vi "FPGA Toggle FPGA LED.vi"() -> ()   [LabVIEW 2011]
uses:
  <vilib>/rvi/eio/common/nirviEmuTemplateMethod_errors.vi
  <vilib>/eio/EIONode/EIONode.xnode
panel:
  in  "FPGA LED period (ms)":u32=500
  out "FPGA LED":bool
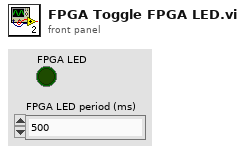
[diagram p1: front panel]
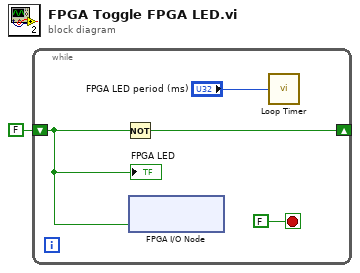
[diagram p0: block diagram]
diagram:
  n1 = while {
    shift-right: [w2] -> _
    shift-left: FALSE -> [w5]
    stop <- FALSE stop-if-true
    n2 = Not(x=w5) -> (.not. x?=w2:bool)
    n3 = xnode "FPGA I/O Node"("FPGA LED"=w5) -> ()  [unwired: 1 in, 1 out]
    n4 = call "Loop Timer"("Count(mSec)"="FPGA LED period (ms)") -> ()  [unwired: 1 out]
    "FPGA LED" <- w5
  }
